vi "change channel metadata.vi"(7 "owner ID":string, 8 "error in":errorcluster, 9 "metadata":string, 10 "channel name":string, 11 "engine configuration in":refnum<class "base TBM sequencer configuration.lvclass">) -> (0 "error out":errorcluster, 3 "engine configuration out":refnum<class "base TBM sequencer configuration.lvclass">)   [LabVIEW 2014, in "base TBM sequencer configuration.lvclass"]
uses:
  base TBM sequencer configuration.lvclass
  <vilib>/NI/Tag Bus/tag/tag descriptor.lvclass
  <vilib>/NI/Tag Bus/tag/tag descriptor.lvclass/tag descriptor.ctl
  base TBM sequencer configuration.lvclass/base TBM sequencer configuration.ctl
  <vilib>/NI/Tag Bus/tag/write metadata.vi
  <vilib>/NI/Tag Bus/tag/write tag name.vi
  <vilib>/NI/Tag Bus Module Framework/channel/TBM channel.lvclass
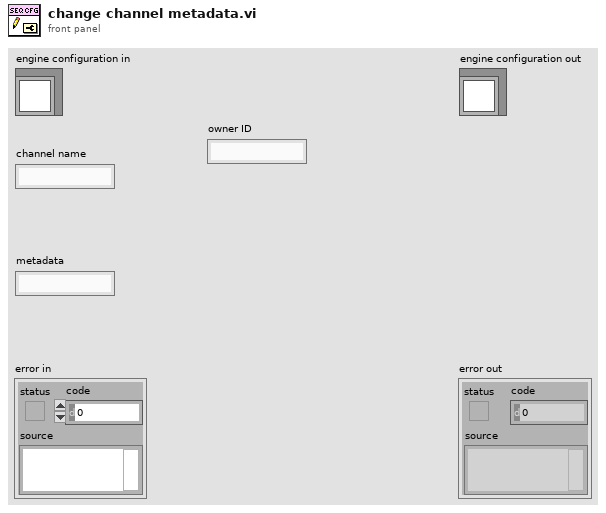
[diagram p1: front panel]
types:
  T1 = typedef "base TBM sequencer configuration.lvclass/Tag Info.ctl" = cluster{"Channel":refnum<class "TBM channel.lvclass">, "Writers":string[], "Readers":string[], "Owning ID":string}
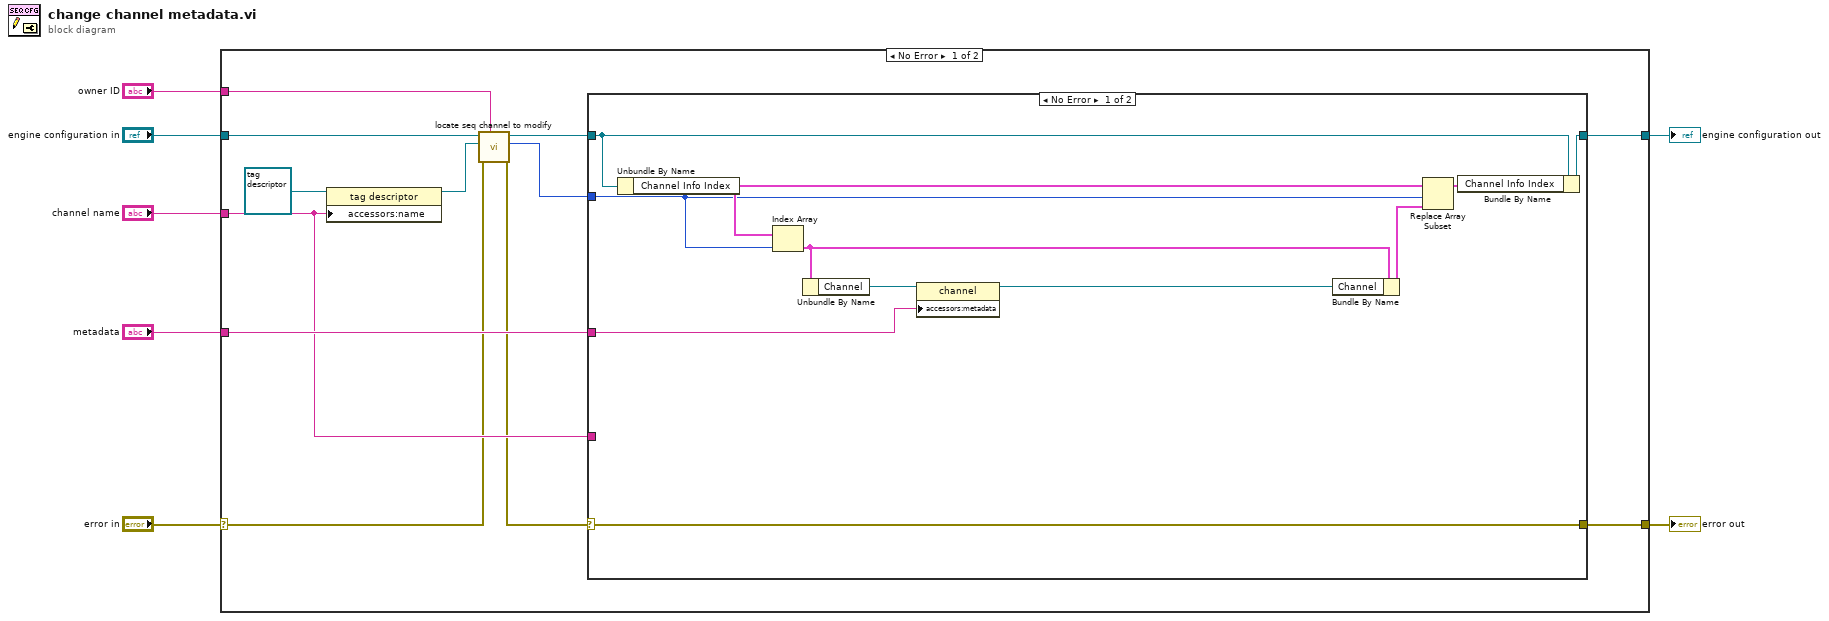
[diagram p0: block diagram]
diagram:
  n1 = case shown="No Error" "error in" {
    selector: "error in" -> [w10 w34]
    tunnel: [w17 w34] -> w6
    tunnel: [w18 w33] -> w4
    tunnel: "engine configuration in" -> [w14 w33]
    tunnel: "channel name" -> [w15 _]
    tunnel: "metadata" -> [w16 _]
    tunnel: "owner ID" -> [w11 _]
    frame No Error {
      n2 = property class="tag descriptor"(reference=refnum<class "tag descriptor.lvclass"> refnum ("tag descriptor"), "accessors:name"=w15) -> (reference out=w12:refnum<class "tag descriptor.lvclass">)  [unwired: 1 in, 1 out]
      n3 = call "locate seq channel to modify.vi"("owner ID"=w11, "error in"=w10, "tag descriptor"=w12, "engine configuration in"=w14) -> ("error out"=w9:errorcluster, "index"=w8:i32, "engine configuration out"=w13:refnum<class "base TBM sequencer configuration.lvclass">)  [unwired: 5 in]
      n4 = case shown="No Error" w9 {
        selector: w9 -> [w20 w31]
        tunnel: w13 -> [w22 w32]
        tunnel: [w23 w32] -> w18
        tunnel: [w20 w31] -> w17
        tunnel: w16 -> [w29 _]
        tunnel: w15 -> [_ _]
        tunnel: w8 -> [w21 _]
        frame No Error {
          n5 = Unbundle By Name(w22) -> ("Channel Info Index"=w26:T1[])
          n6 = Index Array(array=w26, index=w21) -> (element=w28:T1)
          n7 = Unbundle By Name(w28) -> ("Channel"=w30:refnum<class "TBM channel.lvclass">)
          n8 = property class="channel"(reference=w30, "accessors:metadata"=w29) -> (reference out=w27:refnum<class "TBM channel.lvclass">)  [unwired: 1 in, 1 out]
          n9 = Bundle By Name(cluster=w28, "Channel"=w27) -> (w25:T1)
          n10 = Replace Array Subset(array=w26, new element=w25, index=w21) -> (w24:T1[])
          n11 = Bundle By Name(cluster=w22, "Channel Info Index"=w24) -> (w23:refnum<class "base TBM sequencer configuration.lvclass">)
        }
        frame Error {
        }
      }
    }
    frame Error {
    }
  }
  "error out" <- w6
  "engine configuration out" <- w4
